vi "CreateCSV.vi"() -> ()   [LabVIEW 2020]
uses:
  <vilib>/Utility/file.llb/Write Delimited Spreadsheet (string).vi
panel:
  in  "Table Control":string[][](table)=[["Name", "Age", "Salary", "Gender"], ["Sanket Shende", "19", "100000", "Male"], ["Jegatha B", "19", "100000", "Female"]]
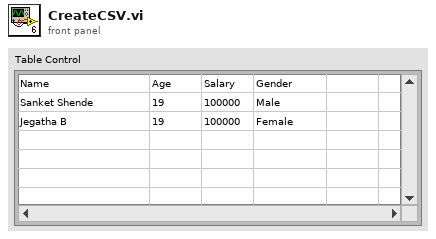
[diagram p1: front panel]
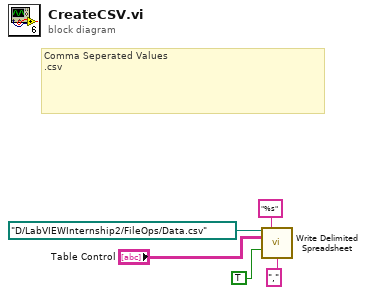
[diagram p0: block diagram]
diagram:
  # "Comma Seperated Values\n.csv"
  n1 = call-poly <vilib>:"Write Delimited Spreadsheet.vi"("file path (dialog if empty)"=path "D:/LabVIEWInternship2/FileOps/Data.csv", "format (%s)"="%s", "2D data"="Table Control", "append to file? (new file:F)"=TRUE, "delimiter (\\t)"="," ("delimiter (\\t)")) -> ()  [unwired: 9 in, 2 out]
